vi "Flatten.vi"(8 "error in":errorcluster, 9 "Data":T1) -> (0 "error out":errorcluster, 2 "Buffer":u8[](array[numeric]) format="%.0x")   [LabVIEW 2020, in "Events.lvlib"]
uses:
  Events.lvlib
  Data.ctl
  Event/Event.lvlib
  Error/Data.ctl
  Error/Error.lvlib
  EventLevel/Enumeration.ctl
  EventLevel/EventLevel.lvlib
  Event/Data.ctl
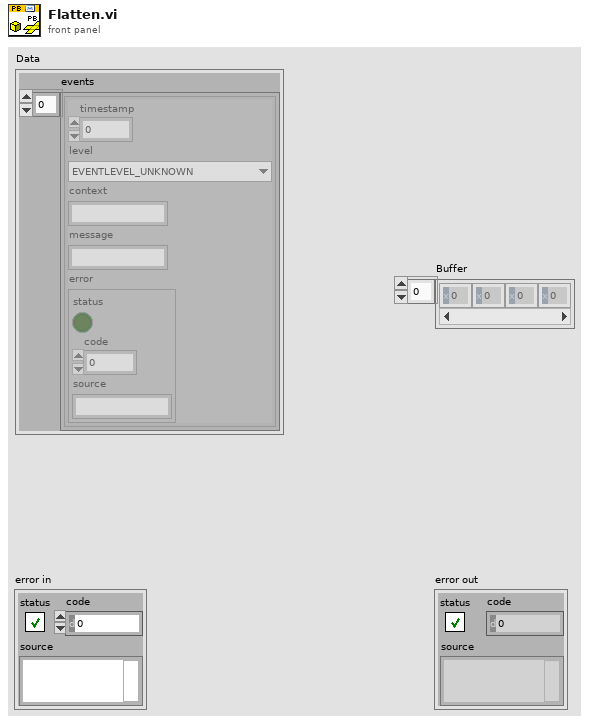
[diagram p1: front panel]
types:
  T1 = typedef "Events.lvlib/Data.ctl" = cluster{"events":T2[]}
  T2 = typedef "Event.lvlib/Data.ctl" = cluster{"timestamp":i64, "level":T3, "context":string, "message":string, "error":T4}
  T3 = typedef "EventLevel.lvlib/Enumeration.ctl" = enum16{"EVENTLEVEL_UNKNOWN", "EVENTLEVEL_DEBUG", "EVENTLEVEL_INFO", "EVENTLEVEL_WARNING", "EVENTLEVEL_ERROR"}
  T4 = typedef "Error.lvlib/Data.ctl" = errorcluster
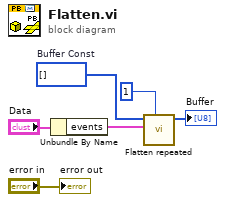
[diagram p0: block diagram]
diagram:
  w4 = u8[] []  # Buffer Const
  n1 = Unbundle By Name("Data") -> ("events"=w3:T2[])
  n2 = call "Flatten repeated.vi"("Field Number"=1, "Data"=w3, "Buffer in"=w4) -> ("Buffer"=→"Buffer":u8[])  [unwired: 8 in]
  "error out" <- "error in"
